vi "TreeTraversal.vi"() -> ()   [LabVIEW 2022 SP3, in "TreeTraversal.lvlib"]
uses:
  TreeTraversal.lvlib
  Public/Classes/IDevice/IDevice.lvclass
  Public/Classes/daqUtils/daqUtils.lvlib
  Public/Classes/daqUtils/Tree/Tree.lvlib
  Public/Classes/IInstance/IInstance.lvclass
panel:
  in  "Tree":string(tree)
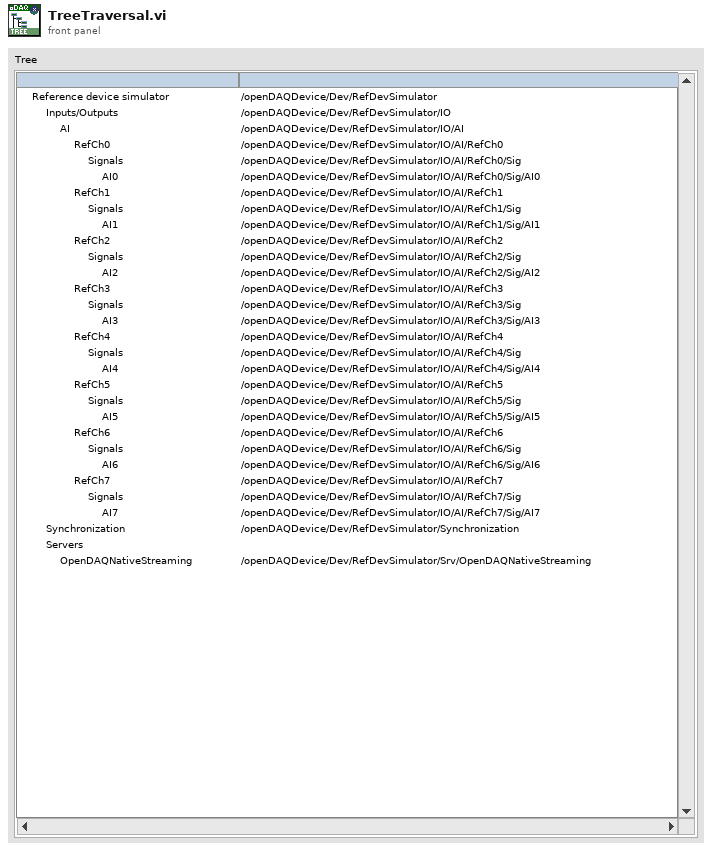
[diagram p1: front panel]
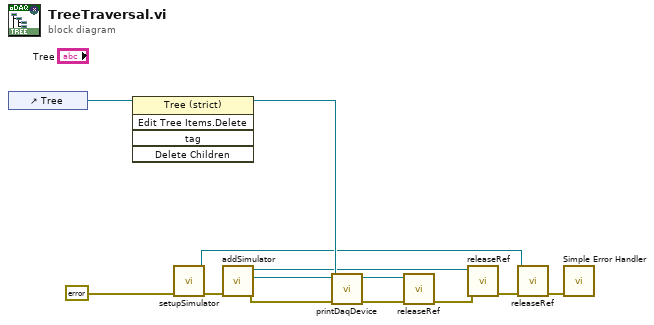
[diagram p0: block diagram]
diagram:
  n1 = control-ref of="Tree"() -> (w6:refnum<vi>)
  n2 = invoke class="Tree (strict)" method="Edit Tree Items.Delete"(reference=w6) -> (reference out=w13:refnum<vi>)  [unwired: 4 in, 4 out]
  n3 = call "setupSimulator.vi"("error in (no error)"=errorcluster {"status"=FALSE, "code"=0, "source"=""}) -> ("error out"=w4:errorcluster, "IInstance out"=w1:refnum<class "IInstance.lvclass">)  [unwired: 9 in]
  n4 = call "addSimulator.vi"("error in (no error)"=w4) -> ("error out"=w11:errorcluster, "IDevice out"=w12:refnum<class "IDevice.lvclass">, "IInstance out"=w8:refnum<class "IInstance.lvclass">)  [unwired: 8 in]
  n5 = call "printDaqDevice.vi"("error in"=w11, "TreeRef"=w13, "baseObject in"=w12) -> ("error out"=w9:errorcluster, "baseObject out"=w10:refnum<class "IDevice.lvclass">)  [unwired: 7 in]
  n6 = call-dynamic "releaseRef.vi"("error in (no error)"=w9, "IBaseObject in"=w10) -> ("error out"=w7:errorcluster)  [unwired: 9 in]
  n7 = call-dynamic "releaseRef.vi"("error in (no error)"=w7, "IBaseObject in"=w8) -> ("error out"=w3:errorcluster)  [unwired: 9 in]
  n8 = call-dynamic "releaseRef.vi"("error in (no error)"=w3, "IBaseObject in"=w1) -> ("error out"=w2:errorcluster)  [unwired: 9 in]
  n9 = call <vilib>:"Simple Error Handler.vi"("error in (no error)"=w2) -> ()  [unwired: 4 in, 5 out]
